vi "Pump Start Detector (TI_PSA).vi"(0 "Arm Level":i32, 2 "Level":i32, 5 "Disarm Level":i32, 7 "Spike Window":i32, 9 "Min Window":i32, 11 "Max Window":i32, 13 "Reset":bool) -> (4 "Restarts":u32)   [LabVIEW 2019]
uses:
  <vilib>/rvi/Emulation/niFpgaGetClockAttributes.vi
  <vilib>/rvi/Emulation/niFpgaSctlEmulationGetInTimedLoop.vi
  <vilib>/rvi/Emulation/niFpgaEmulationReportErrorSimple.vi
  <vilib>/rvi/Emulation/niFpgaCriticalErrorInLSC.vi
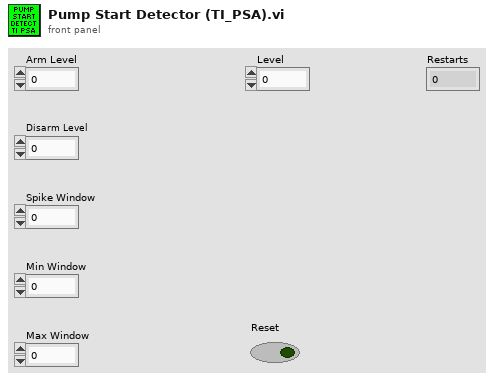
[diagram p1: front panel]
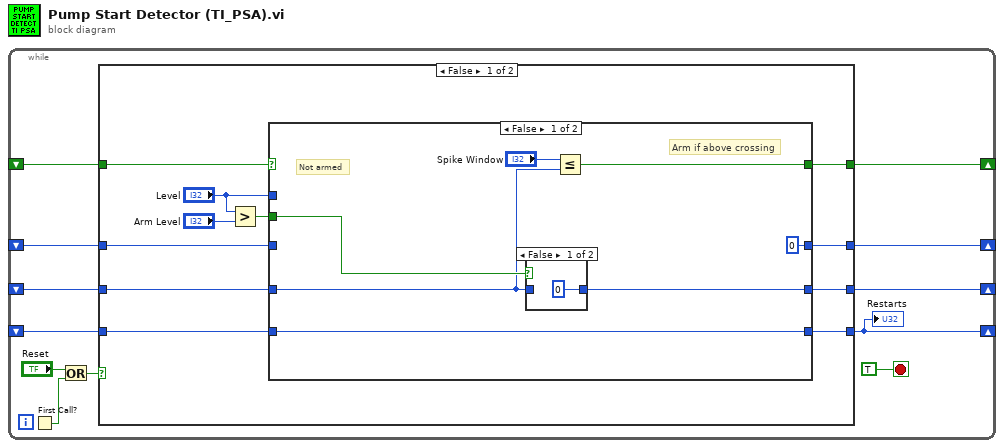
[diagram p0: block diagram]
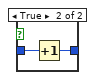
[diagram p2: hidden frame]
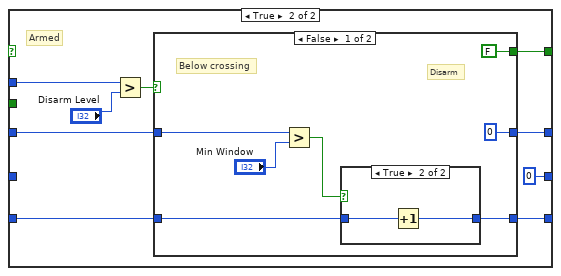
[diagram p3: hidden frame]
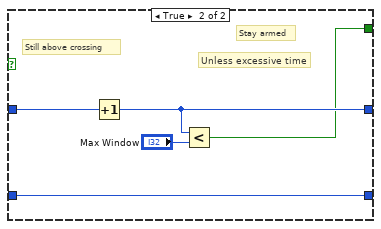
[diagram p5: hidden frame]
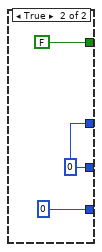
[diagram p6: hidden frame]
diagram:
  n1 = while {
    shift-right: [w3] -> _
    shift-left: _ -> [w6]
    shift-right: [w5] -> _
    shift-left: _ -> [w7]
    shift-right: [w4] -> _
    shift-left: _ -> [w8]
    shift-right: [w2] -> _
    shift-left: _ -> [w1]
    stop <- TRUE stop-if-true
    n2 = First Call?() -> (First Call?: T/F=w10:bool)
    n3 = Or(x="Reset", y=w10) -> (x .or. y?=w9:bool)
    n4 = case shown="False" w9 {
      tunnel: w8 -> [w19 _]
      tunnel: w7 -> [w18 _]
      tunnel: w6 -> [w21 _]
      tunnel: [w20 u32 0 ("Restarts")] -> w3
      tunnel: [w22 w58] -> w5
      tunnel: [w23 FALSE] -> w4
      tunnel: [w17 w58] -> w2
      tunnel: w1 -> [w16 _]
      frame False {
        n5 = Greater?(x="Level", y="Arm Level") -> (0:w13:bool)
        n6 = case shown="False" w19 {
          tunnel: [w27 w40] -> w23
          tunnel: [0 ("Restarts") w41] -> w22
          tunnel: [w29 w38] -> w20
          tunnel: w21 -> [w29 w39]
          tunnel: w13 -> [w26 _]
          tunnel: w18 -> [_ w42]
          tunnel: "Level" -> [_ w35]
          tunnel: [w24 0] -> w17
          tunnel: w16 -> [w25 _]
          frame False {
            # "Arm if above crossing"
            # "Not armed"
            n7 = case shown="False" w26 {
              tunnel: w25 -> [_ w33]
              tunnel: [0 w32] -> w24
              frame False {
              }
              frame True {
                n8 = Increment(x=w33) -> (x+1=w32:i32)
              }
            }
            n9 = Less Or Equal?(x="Spike Window", y=w25) -> (x <= y?=w27:bool)
          }
          frame True {
            # "Armed"
            n10 = Greater?(x=w35, y="Disarm Level") -> (0:w36:bool)
            n11 = case shown="False" w36 {
              tunnel: w42 -> [w43 w57]
              tunnel: [0 ("Restarts") w55] -> w41
              tunnel: [FALSE w53] -> w40
              tunnel: w39 -> [w45 w56]
              tunnel: [w44 w56] -> w38
              frame False {
                # "Disarm"
                # "Below crossing"
                n12 = Greater?(x=w43, y="Min Window") -> (0:w46:bool)
                n13 = case shown="True" w46 {
                  tunnel: w45 -> [w50 w52]
                  tunnel: [w50 w51] -> w44
                  frame False {
                  }
                  frame True {
                    n14 = Increment(x=w52) -> (x+1=w51:u32)
                  }
                }
              }
              frame True {
                # "Unless excessive time"
                # "Stay armed"
                # "Still above crossing"
                n15 = Increment(x=w57) -> (x+1=w55:i32)
                n16 = Less?(x=w55, y="Max Window") -> (x < y?=w53:bool)
              }
            }
          }
        }
      }
      frame True {
        w58 = 0
      }
    }
    "Restarts" <- w3
  }
